vi "Compile - Rx Buffered Channel Refs.vi"(6 "Packet Name":string, 8 "error in (no error)":errorcluster, 11 "Item Ref in":T1 format="%.0x") -> (0 "error out":errorcluster, 3 "Item Ref out":T1 format="%.0x", 4 "Tx Ref Array":T2(array[cluster]) {"VS Refs" format="%.0x"})   [LabVIEW 2016, in "UDP-Custom-Device System Explorer.lvlib"]
uses:
  UDP-Custom-Device System Explorer.lvlib
  <vilib>/NI Veristand/Custom Device API/Custom Device Item Ref.ctl
  <vilib>/NI VeriStand/Custom Device API/Custom Device API.lvlib
  Property Accessors/Buffered Data Packet.lvlib
  <vilib>/NI VeriStand/Custom Device Tools/Custom Device Utility Library/Custom Device Utility Library.lvlib
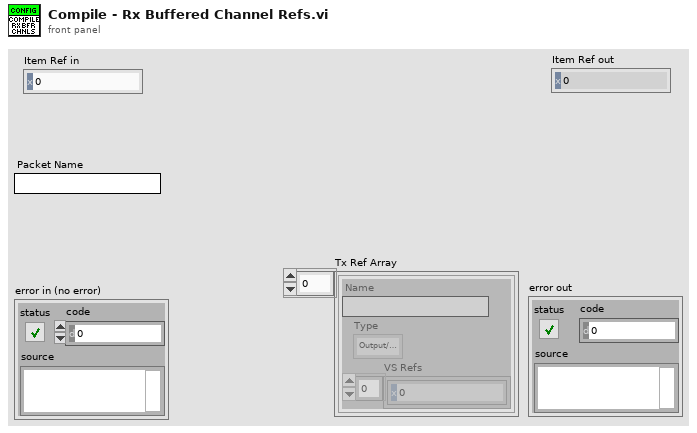
[diagram p1: front panel]
types:
  T1 = typedef "Custom Device API.lvlib/Custom Device Item Ref.ctl" = u64
  T2 = cluster{"Name":string, "Type":enum16{"Output/Write", "Input/Read", "Input/ReadWrite"}, "VS Refs":T1[]}[]
  T3 = enum16{"Output/Write", "Input/Read", "Input/ReadWrite"}
  T4 = cluster{"Name":string, "Type":enum16{"Output/Write", "Input/Read", "Input/ReadWrite"}, "VS Refs":T1[]}
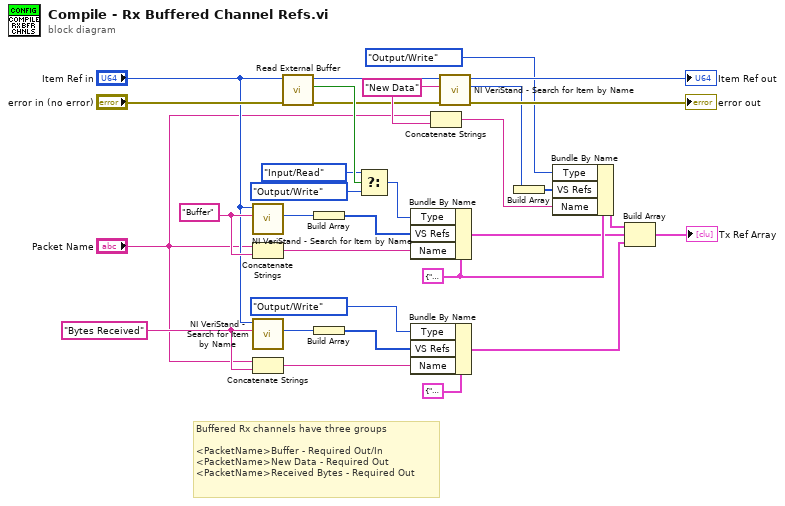
[diagram p0: block diagram]
diagram:
  w5 = "Bytes Received" ("Item GUID")
  w14 = "New Data" ("Item GUID")
  w11 = "Buffer" ("Item GUID")
  w18 = T4 {"Name"="", "Type"=enum."Output/Write", "VS Refs"=[]} ("Group")
  # "Buffered Rx channels have three groups\n\n<PacketName>Buffer - Required Out/In\n<PacketName>New Data - Required Out\n<PacketName>Received Bytes - Required Out"
  n1 = call <vilib>:"NI VeriStand - Search for Item by Name.vi"("Item Name"=w11, "Section Ref in"="Item Ref in") -> ("Item Ref"=w10:T1)  [unwired: 6 in, 3 out]
  n2 = Concatenate Strings("Packet Name", w11) -> (w27:string)
  n3 = call <vilib>:"NI VeriStand - Search for Item by Name.vi"("Item Name"=w5, "Section Ref in"="Item Ref in") -> ("Item Ref"=w9:T1)  [unwired: 6 in, 3 out]
  n4 = Concatenate Strings("Packet Name", w5) -> (w6:string)
  n5 = call "Read External Buffer.vi"("error in (no error)"="error in (no error)", "Node Ptr"="Item Ref in") -> ("error out"=w13:errorcluster, "External Buffer"=w25:bool, "Node Ptr out"=w15:T1)  [unwired: 7 in]
  n6 = Build Array(w10) -> (w26:T1[])
  n7 = Build Array(w9) -> (w7:T1[])
  n8 = Select(t=T3."Input/Read" ("Type"), s=w25, f=T3."Output/Write" ("Type")) -> (s? t:f=w22:T3)
  n9 = Bundle By Name(cluster=w18, "Type"=w22, "VS Refs"=w26, "Name"=w27) -> (w16:T4)
  n10 = Bundle By Name(cluster=T4 {"Name"="", "Type"=enum."Output/Write", "VS Refs"=[]} ("Group"), "Type"=T3."Output/Write", "VS Refs"=w7, "Name"=w6) -> (w2:T4)
  n11 = Concatenate Strings("Packet Name", w14) -> (w19:string)
  n12 = call <vilib>:"NI VeriStand - Search for Item by Name.vi"("error in"=w13, "Item Name"=w14, "Section Ref in"=w15) -> ("error out"=→"error out":errorcluster, "Item Ref"=w12:T1, "Section Ref out"=→"Item Ref out":T1)  [unwired: 5 in, 1 out]
  n13 = Build Array(w12) -> (w20:T1[])
  n14 = Bundle By Name(cluster=w18, "Type"=T3."Output/Write", "VS Refs"=w20, "Name"=w19) -> (w17:T4)
  n15 = Build Array(w17, w16, w2) -> (→"Tx Ref Array":T2)
